vi "HB_ThreadPool.MainLoopingTask.vi"() -> ()   [LabVIEW 2009, in "HB_BaseClass_Examples.lvlib"]
doc: "Simple application to test the HGF_ThreadPool with a simple class."
uses:
  HB_BaseClass_Examples.lvlib
  HB_Factory/HB_Factory.lvclass
  lib.lib/HGF_LVC/HGF_BaseClasses/HGF_Factory/HGF_Factory.lvclass
  lib.lib/HGF_LVC/HGF_BaseClasses/HGF_Event/HGF_Event.lvclass
  lib.lib/HGF_LVC/HGF_BaseClasses/HGF_ThreadTask/HGF_ThreadTask.lvclass
  HB_Simple/Visitors/Increment/HB_Simple_Increment.lvclass
  HB_Simple/HB_Simple.lvclass
  lib.lib/HGF_LVC/HGF_BaseClasses/HGF_Queue/HGF_Queue.lvclass
  lib.lib/HGF_LVC/HGF_BaseClasses/HGF_Visitable/HGF_Visitable.lvclass
  lib.lib/HGF_LVC/HGF_BaseClasses/HGF_Stop/HGF_Stop.lvclass
  lib.lib/HGF_LVC/HGF_BaseClasses/HGF_ThreadPool/HGF_ThreadPool.lvclass
  lib.lib/HGF_LVC/HGF_BaseClasses/HGF_Reference/HGF_Reference.lvclass
  lib.lib/HGF_LVC/HGF_Auxiliary/HGF_Auxiliary.lvlib
  lib.lib/HGF_LVC/HGF_BaseClasses/HGF_Timing/HGF_Timing.lvclass
panel:
  in  "Decrement":bool
  out "objectName":string
  in  "nofObjects":i32=10
  out "Waveform Chart":dbl(graph)
  in  "timeout in ms (-1)":i32=3000
  out "nofTasksInQueueOut":i32
  out "nofTasksWaiting":i32
  out "autoIncrementLimit":i32=-1
  out "nofThreads":i32
  out "Default Destination timed out?":bool
  out "got object?":bool
  out "error":errorcluster
  in  "stop":bool
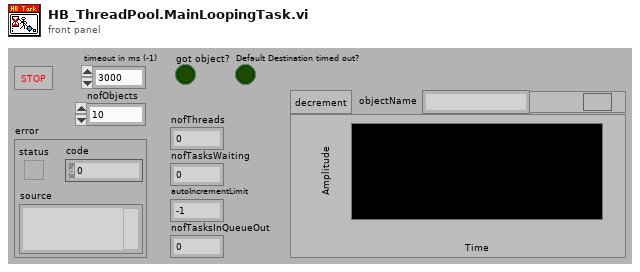
[diagram p1: front panel]
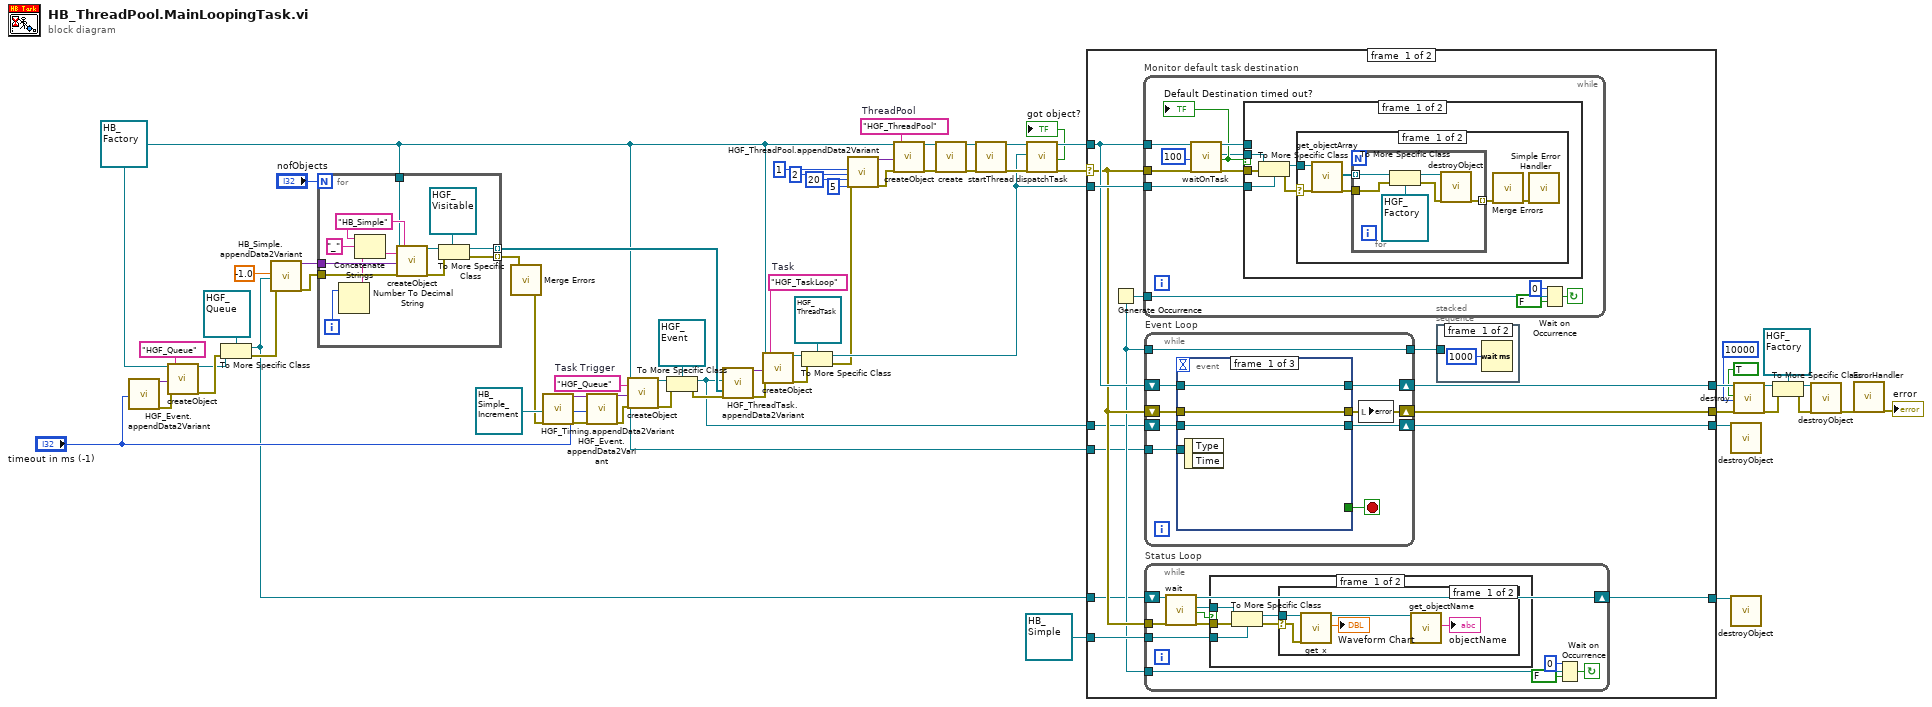
[diagram p0: block diagram]
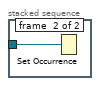
[diagram p2: hidden frame]
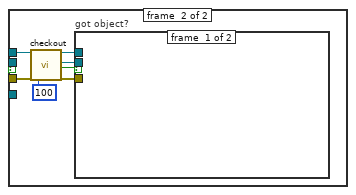
[diagram p6: hidden frame]
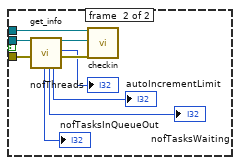
[diagram p7: hidden frame]
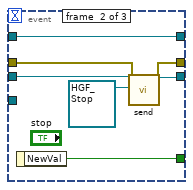
[diagram p8: hidden frame]
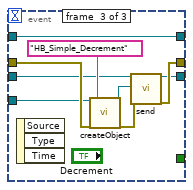
[diagram p9: hidden frame]
diagram:
  w48 = "HGF_Queue"  # Task Trigger
  w47 = "HGF_TaskLoop"  # Task
  w39 = "HGF_ThreadPool"  # ThreadPool
  w1 = refnum<class "HB_Factory.lvclass"> refnum ("HB_Factory.lvclass")
  n1 = call "HGF_Event.appendData2Variant.vi"("timeout in ms (-1)"="timeout in ms (-1)") -> ("dup initData"=w21:variant, "error out"=w22:errorcluster)  [unwired: 2 in, 15 out]
  n2 = call "createObject.vi"("HGF_Factory"=w1, "initializationData"=w21, "error in (no error)"=w22, "className"="HGF_Queue") -> ("HGF_Object"=w18:refnum<class "HGF_Factory.lvclass">, "error out"=w19:errorcluster)  [unwired: 2 in, 12 out]
  n3 = To More Specific Class(target class=refnum<class "HGF_Queue.lvclass"> refnum ("HGF_BaseClasses.lvlib:HGF_Queue.lvclass"), reference=w18, error in=w19) -> (specific class reference=w11:refnum<class "HGF_Queue.lvclass">, error out=w12:errorcluster)
  n4 = call "HB_Simple.appendData2Variant.vi"("x"=-1.0, "statusEvent"=w11, "error in (no error)"=w12) -> ("dup initData"=w14:variant, "error out"=w13:errorcluster)  [unwired: 15 in]
  n5 = for {
    N: "nofObjects" -> [_]
    tunnel: [w69] -> w36 mode=indexing
    tunnel: w1 -> [w74]
    tunnel: [w73] -> w8 mode=indexing
    tunnel: w14 -> [w71]
    tunnel: w13 -> [w70]
    i -> [w68]
    w77 = "HB_Simple" ("className")
    n6 = Number To Decimal String(number=w68) -> (decimal integer string=w67:string)  [unwired: 1 out]
    n7 = Concatenate Strings(w77, "_" ("string"), w67) -> (w75:string)
    n8 = call "createObject.vi"("HGF_Factory"=w74, "objectName"=w75, "initializationData"=w71, "error in (no error)"=w70, "className"=w77) -> ("HGF_Object"=w78:refnum<class "HGF_Factory.lvclass">, "error out"=w79:errorcluster)  [unwired: 1 in, 12 out]
    n9 = To More Specific Class(target class=refnum<class "HGF_Visitable.lvclass"> refnum ("HGF_BaseClasses.lvlib:HGF_Visitable.lvclass"), reference=w78, error in=w79) -> (specific class reference=w69:refnum<class "HGF_Visitable.lvclass">, error out=w73:errorcluster)
  }
  n10 = call <vilib>:"Merge Errors.vi"("error array in"=w8) -> ("error out"=w7:errorcluster)  [unwired: 3 in, 3 out]
  n11 = call "HGF_Timing.appendData2Variant.vi"("defaultObject"=refnum<class "HB_Simple_Increment.lvclass"> refnum ("HGF_BaseClass_Examples.lvlib:HB_Simple_Increment.lvclass"), "error in (no error)"=w7) -> ("dup initData"=w26:variant, "error out"=w25:errorcluster)  [unwired: 1 in, 15 out]
  n12 = call "HGF_Event.appendData2Variant.vi"("initData"=w26, "timeout in ms (-1)"="timeout in ms (-1)", "error in (no error)"=w25) -> ("dup initData"=w53:variant, "error out"=w52:errorcluster)  [unwired: 1 in, 14 out]
  n13 = call "createObject.vi"("HGF_Factory"=w1, "initializationData"=w53, "error in (no error)"=w52, "className"=w48) -> ("HGF_Object"=w45:refnum<class "HGF_Factory.lvclass">, "error out"=w54:errorcluster)  [unwired: 2 in, 12 out]
  n14 = To More Specific Class(target class=refnum<class "HGF_Event.lvclass"> refnum ("HGF_BaseClasses.lvlib:HGF_Event.lvclass"), reference=w45, error in=w54) -> (specific class reference=w24:refnum<class "HGF_Event.lvclass">, error out=w38:errorcluster)
  n15 = call "HGF_ThreadTask.appendData2Variant.vi"("taskTrigger"=w24, "objectArray"=w36, "error in (no error)"=w38) -> ("dup initData"=w35:variant, "error out"=w34:errorcluster)  [unwired: 3 in, 12 out]
  n16 = call "createObject.vi"("HGF_Factory"=w1, "initializationData"=w35, "error in (no error)"=w34, "className"=w47) -> ("HGF_Object"=w44:refnum<class "HGF_Factory.lvclass">, "error out"=w51:errorcluster)  [unwired: 2 in, 12 out]
  n17 = To More Specific Class(target class=refnum<class "HGF_ThreadTask.lvclass"> refnum ("HGF_BaseClasses.lvlib:HGF_ThreadTask.lvclass"), reference=w44, error in=w51) -> (specific class reference=w27:refnum<class "HGF_ThreadTask.lvclass">, error out=w15:errorcluster)
  n18 = call "HGF_ThreadPool.appendData2Variant.vi"("initialNofThreads (0)"=1 ("initialNofThreads"), "incThreads(1)"=2 ("incThreads"), "maxNofThreads (-1:unlimited)"=20 ("maxNofThreads"), "error in (no error)"=w15, "autoIncrementLimit (-1)"=5) -> ("dup initData"=w65:variant, "error out"=w16:errorcluster)  [unwired: 2 in, 11 out]
  n19 = call "createObject.vi"("HGF_Factory"=w1, "initializationData"=w65, "error in (no error)"=w16, "className"=w39) -> ("HGF_Object"=w46:refnum<class "HGF_Factory.lvclass">, "error out"=w64:errorcluster)  [unwired: 2 in, 12 out]
  n20 = call "create.vi"("Object"=w46, "error in (no error)"=w64) -> ("HGF_Reference"=w66:refnum<class "HGF_Reference.lvclass">, "error out"=w60:errorcluster)  [unwired: 1 in, 15 out]
  n21 = call "startThread.vi"("HGF_ThreadPool_Reference"=w66, "error in (no error)"=w60) -> ("dup HGF_ThreadPool_Reference"=w32:refnum<class "HGF_Reference.lvclass">, "error out"=w30:errorcluster)  [unwired: 1 in, 15 out]
  n22 = call "dispatchTask.vi"("HGF_ThreadPool_Reference"=w32, "HGF_ThreadTask"=w27, "error in (no error)"=w30) -> ("dup HGF_ThreadPool_Reference"=w31:refnum<class "HGF_Reference.lvclass">, "got object?"=→"got object?":bool, "error out"=w29:errorcluster)  [unwired: 1 in, 13 out]
  n23 = case shown="No Error" w29 {
    selector: w29 -> [w87 w191]
    tunnel: w31 -> [w89 w192]
    tunnel: [w92 w192] -> w50
    tunnel: w27 -> [w90 _]
    tunnel: [w91 w191] -> w49
    tunnel: w24 -> [w82 w189]
    tunnel: w11 -> [w83 w190]
    tunnel: refnum<class "HB_Simple.lvclass"> refnum ("HGF_BaseClass_Examples.lvlib:HB_Simple.lvclass") -> [w86 _]
    tunnel: w1 -> [w84 _]
    tunnel: [w81 w190] -> w3
    tunnel: [w80 w189] -> w2
    frame #0 {
      n24 = Generate Occurrence() -> (w85:refnum<k4>)
      n25 = while "Monitor default task destination" {
        tunnel: w90 -> [w123]
        tunnel: w89 -> [w122]
        tunnel: w87 -> [w121]
        tunnel: w85 -> [w116]
        stop <- w117 continue-if-true
        n26 = call "waitOnTask.vi"("HGF_ThreadPool_Reference"=w122, "timeout in ms (-1)"=100, "error in (no error)"=w121) -> ("dup HGF_ThreadPool_Reference"=w127:refnum<class "HGF_Reference.lvclass">, "HGF_Task"=w125:refnum<class "HGF_ThreadTask.lvclass">, "timed out?"=w126:bool, "error out"=w120:errorcluster)  [unwired: 13 out]
        "Default Destination timed out?" <- w126
        n27 = case "timed out?" shown="False" w126 {
          tunnel: w125 -> [w132 _]
          tunnel: w120 -> [w131 w145]
          tunnel: w127 -> [_ w146]
          tunnel: w123 -> [w128 _]
          frame #0 {
            n28 = To More Specific Class(target class=w128, reference=w132, error in=w131) -> (specific class reference=w130:refnum<class "HGF_ThreadTask.lvclass">, error out=w129:errorcluster)
            n29 = case shown="No Error" w129 {
              selector: w129 -> [w137 _]
              tunnel: w130 -> [w138 _]
              frame #0 {
                n30 = call "get_objectArray.vi"("HGF_ThreadTask"=w138, "error in (no error)"=w137) -> ("objectArray"=w133:refnum<class>[], "error out"=w135:errorcluster)  [unwired: 16 out]
                n31 = for {
                  tunnel: w135 -> [w141]
                  tunnel: [w144] -> w136 mode=indexing
                  tunnel: w133 -> [w143] mode=indexing
                  n32 = To More Specific Class(target class=refnum<class "HGF_Factory.lvclass"> refnum ("HGF_BaseClasses.lvlib:HGF_Factory.lvclass"), reference=w143, error in=w141) -> (specific class reference=w142:refnum<class "HGF_Factory.lvclass">, error out=w140:errorcluster)
                  n33 = call "destroyObject.vi"("HGF_Factory"=w142, "error in (no error)"=w140) -> ("error out"=w144:errorcluster)  [unwired: 17 out]
                }
                n34 = call <vilib>:"Merge Errors.vi"("error array in"=w136) -> ("error out"=w134:errorcluster)  [unwired: 3 in, 3 out]
                n35 = call <vilib>:"Simple Error Handler.vi"("error in (no error)"=w134) -> ()  [unwired: 1 in, 8 out]
              }
              frame #1 {
              }
            }
          }
          frame #1 {
            n36 = call "checkout.vi"("HGF_ThreadPool_Reference"=w146, "timeout in ms (-1)"=100, "error in (no error)"=w145) -> ("dup HGF_ThreadPool_Reference"=w147:refnum<class "HGF_Reference.lvclass">, "HGF_ThreadPool"=w148:refnum<class "HGF_ThreadPool.lvclass">, "got object?"=w151:bool, "error out"=w149:errorcluster)  [unwired: 13 out]
            n37 = case "got object?" shown="True" w151 {
              tunnel: w147 -> [_ w160]
              tunnel: w148 -> [_ w159]
              tunnel: w149 -> [_ w158]
              frame #0 {
              }
              frame #1 {
                n38 = call "get_info.vi"("HGF_ThreadPool"=w159, "error in (no error)"=w158) -> ("nofTasksInQueueOut"=→"nofTasksInQueueOut":i32, "nofTasksWaiting"=→"nofTasksWaiting":i32, "autoIncrementLimit"=→"autoIncrementLimit":i32, "dup HGF_ThreadPool"=w156:refnum<class "HGF_ThreadPool.lvclass">, "nofThreads"=→"nofThreads":i32, "error out"=w157:errorcluster)  [unwired: 12 out]
                n39 = call "checkin.vi"("HGF_Reference"=w160, "Object"=w156, "error in (no error)"=w157) -> ()  [unwired: 1 in, 16 out]
              }
            }
          }
        }
        n40 = Wait on Occurrence(1:FALSE ("ignore previous (T)"), 2:w116, 3:0 ("ms timeout (-1)")) -> (0:w117:bool)
      }
      n41 = while "Event Loop" {
        shift-right: [w168] -> w92
        shift-left: w89 -> [w167]
        shift-right: [w164] -> w91
        shift-left: w87 -> [w169]
        tunnel: w85 -> [w163]
        tunnel: [w163] -> w88
        tunnel: w84 -> [w165]
        shift-right: [w161] -> w80
        shift-left: w82 -> [w166]
        stop <- w162 stop-if-true
        n42 = event shown="[1] \"stop\": Value Change" {
          selector: _ -> [_ _ _]
          dyn-events: _ -> [_ _ _]
          timeout: _ -> [_ _ _]
          tunnel: [_ w179 _] -> w162
          tunnel: [w171 w174 w182] -> w164
          tunnel: w169 -> [w171 w175 w186]
          tunnel: [w172 w178 w188] -> w168
          tunnel: w167 -> [w172 w178 w188]
          tunnel: w166 -> [w170 w177 w185]
          tunnel: w165 -> [_ _ w181]
          tunnel: [w170 w173 w180] -> w161
          event #0 {
            n43 = event-data() -> ()  [unwired: 3 out]
          }
          event #1 {
            n44 = event-data() -> ("NewVal"=w179:bool)  [unwired: 1 out]
            n45 = call-dynamic "send.vi"("HGF_Event"=w177, "Object"=refnum<class "HGF_Stop.lvclass"> refnum ("HGF_BaseClasses.lvlib:HGF_Stop.lvclass"), "error in (no error)"=w175) -> ("dup HGF_Event"=w173:refnum<class "HGF_Event.lvclass">, "error out"=w174:errorcluster)  [unwired: 2 in, 13 out]
          }
          event #2 {
            n46 = event-data() -> ()  [unwired: 4 out]
            n47 = call "createObject.vi"("HGF_Factory"=w181, "error in (no error)"=w186, "className"="HB_Simple_Decrement") -> ("HGF_Object"=w184:refnum<class "HGF_Factory.lvclass">, "error out"=w183:errorcluster)  [unwired: 3 in, 12 out]
            n48 = call-dynamic "send.vi"("HGF_Event"=w185, "Object"=w184, "error in (no error)"=w183) -> ("dup HGF_Event"=w180:refnum<class "HGF_Event.lvclass">, "error out"=w182:errorcluster)  [unwired: 2 in, 13 out]
          }
        }
        n49 = local write "error"(w164) -> ()
      }
      n50 = while "Status Loop" {
        tunnel: w87 -> [w104]
        tunnel: w86 -> [w101]
        tunnel: w85 -> [w96]
        shift-right: [w95] -> w81
        shift-left: w83 -> [w105]
        stop <- w97 continue-if-true
        n51 = call-dynamic "wait.vi"("HGF_Queue"=w105, "error in (no error)"=w104) -> ("dup HGF_Queue"=w95:refnum<class "HGF_Queue.lvclass">, "Object"=w102:refnum<class>, "timed out"=w100:bool, "error out"=w103:errorcluster)  [unwired: 2 in, 12 out]
        n52 = case shown="False" w100 {
          tunnel: w103 -> [w110 _]
          tunnel: w102 -> [w109 _]
          tunnel: w101 -> [w108 _]
          frame #0 {
            n53 = To More Specific Class(target class=w108, reference=w109, error in=w110) -> (specific class reference=w106:refnum<class "HB_Simple.lvclass">, error out=w107:errorcluster)
            n54 = case shown="No Error" w107 {
              selector: w107 -> [w114 _]
              tunnel: w106 -> [w115 _]
              frame #0 {
                n55 = call "get_x.vi"("HB_Simple"=w115, "error in (no error)"=w114) -> ("dup HB_Simple"=w112:refnum<class "HB_Simple.lvclass">, "x"=→"Waveform Chart":dbl)  [unwired: 16 out]
                n56 = call "get_objectName.vi"("HGF_Factory"=w112) -> ("objectName"=→"objectName":string)  [unwired: 1 in, 17 out]
              }
              frame #1 {
              }
            }
          }
          frame #1 {
          }
        }
        n57 = Wait on Occurrence(1:FALSE ("ignore previous (T)"), 2:w96, 3:0 ("ms timeout (-1)")) -> (0:w97:bool)
      }
      n58 = stacked-sequence {
        tunnel: w88 -> [_ w94]
        frame #0 {
          n59 = Wait (ms)(milliseconds to wait=u32 1000) -> ()  [unwired: 1 out]
        }
        frame #1 {
          n60 = Set Occurrence(w94) -> ()
        }
      }
    }
    frame #1 {
    }
  }
  n61 = call "destroyObject.vi"("HGF_Factory"=w2) -> ()  [unwired: 1 in, 18 out]
  n62 = call "destroyObject.vi"("HGF_Factory"=w3) -> ()  [unwired: 1 in, 18 out]
  n63 = call "destroy.vi"("HGF_Reference"=w50, "wait for activity? (F)"=TRUE, "timeout /ms (-1)"=10000, "error in (no error)"=w49) -> ("Object"=w59:refnum<class>, "error out"=w57:errorcluster)  [unwired: 14 out]
  n64 = To More Specific Class(target class=refnum<class "HGF_Factory.lvclass"> refnum ("HGF_BaseClasses.lvlib:HGF_Factory.lvclass"), reference=w59, error in=w57) -> (specific class reference=w58:refnum<class "HGF_Factory.lvclass">, error out=w56:errorcluster)
  n65 = call "destroyObject.vi"("HGF_Factory"=w58, "error in (no error)"=w56) -> ("error out"=w37:errorcluster)  [unwired: 17 out]
  n66 = call "ErrorHandler.vi"("error in (no error)"=w37) -> ("error out"=→"error":errorcluster)  [unwired: 6 in, 12 out]
